vi "GenNet Send UDP Message.vi"(5 "Multicast IP Address":string, 6 "timeout [ms]":i32=100, 7 "Receiver Port":u16, 8 "error in (no error)":errorcluster, 10 "Message Data":variant, 11 "UDP Network Connection in":refnum<k16>) -> (0 "error out":errorcluster, 3 "UDP Network Connection out":refnum<k16>)   [LabVIEW 2014, in "hse-gennet.lvlib"]
doc: "Sends a message via TCP/IP to a GenNet-Server module. \n\nThe message is flattened to a string, and the length of the string is prepended before sending it over the network.\n\n____\nHAMPEL SOFTWARE ENGINEERING v0.7.0 (2018-07-16 18:12)"
uses:
  hse-gennet.lvlib
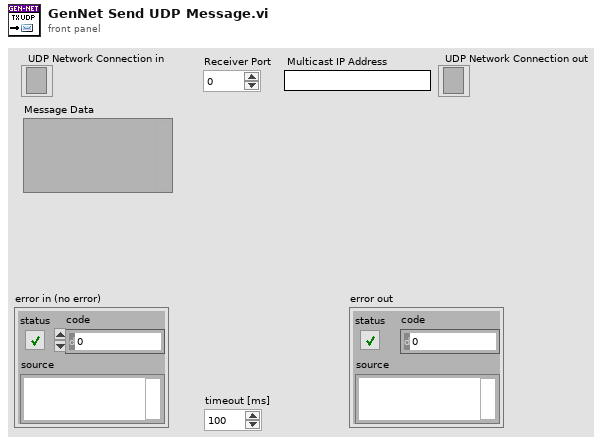
[diagram p1: front panel]
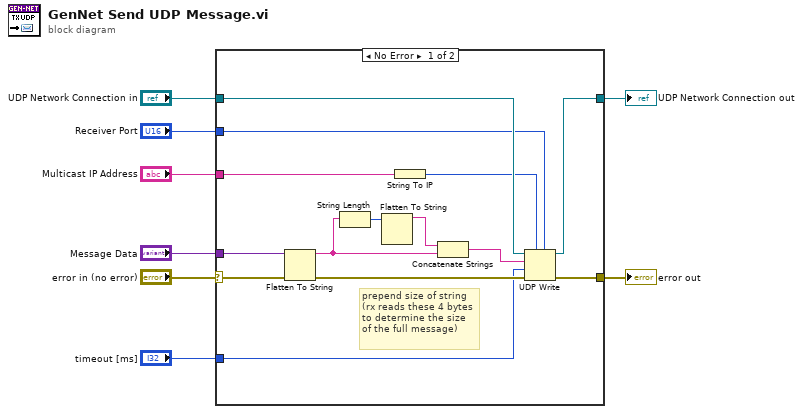
[diagram p0: block diagram]
diagram:
  n1 = case shown="No Error" "error in (no error)" {
    selector: "error in (no error)" -> [w20 w23]
    tunnel: "UDP Network Connection in" -> [w17 w24]
    tunnel: [w14 w23] -> w8
    tunnel: [w16 w24] -> w3
    tunnel: "Message Data" -> [w19 _]
    tunnel: "timeout [ms]" -> [w13 _]
    tunnel: "Multicast IP Address" -> [w10 _]
    tunnel: "Receiver Port" -> [w9 _]
    frame No Error {
      # "prepend size of string\n(rx reads these 4 bytes\nto determine the size\nof the full message)"
      n2 = Flatten To String(anything=w19, error in (no error)=w20) -> (data string=w18:string, error out=w15:errorcluster)  [unwired: 2 in, 1 out]
      n3 = String Length(string=w18) -> (length=w21:i32)
      n4 = Flatten To String(anything=w21) -> (data string=w22:string)  [unwired: 3 in, 2 out]
      n5 = String To IP(1:w10) -> (0:w11:u32)
      n6 = Concatenate Strings(w22, w18) -> (w12:string)
      n7 = UDP Write(address=w11, port or service name=w9, connection ID=w17, data in=w12, 8:w15, 9:w13) -> (error out=w14:errorcluster, 3:w16:refnum<k16>)
    }
    frame Error {
    }
  }
  "error out" <- w8
  "UDP Network Connection out" <- w3
